vi "7.vi"() -> ()   [LabVIEW 2017]
uses:
  <vilib>/Utility/file.llb/Write Delimited Spreadsheet (DBL).vi
  <vilib>/measure/NI_MABase.lvlib
panel:
  out "Array":dbl[][](array[numeric]) caption="数组"
  out "波形图":waveform(dbl)(graph)
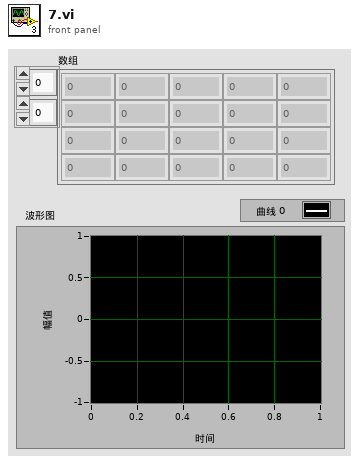
[diagram p1: front panel]
types:
  T1 = enum16{"open", "replace", "create", "open or create", "replace or create", "replace or create with confirmation"}
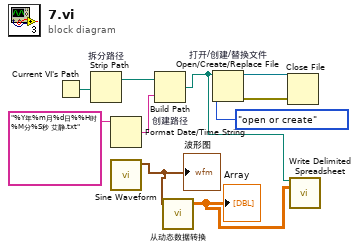
[diagram p0: block diagram]
diagram:
  n1 = Current VI's Path() -> (path=w9:path)
  n2 = Strip Path "拆分路径"(path=w9) -> (stripped path=w7:path)  [unwired: 1 out]
  n3 = Format Date/Time String(time format string (%c)="%Y年%m月%d日%%H时%M分%S秒 艾静.txt" ("时间格式字符串(%c)")) -> (date/time string=w8:string)  [unwired: 2 in]
  n4 = call <vilib>:"Sine Waveform.vi"() -> ("signal out"=w5:waveform(dbl))  [unwired: 10 in, 1 out]
  "波形图" <- w5
  n5 = Build Path "创建路径"(base path=w7, name or relative path=w8) -> (appended path=w3:path)
  n6 = call "从动态数据转换"("Dynamic Data Type"=w5) -> ("Array"=w4:dbl[][])  [unwired: 3 in]
  "Array" <- w4
  n7 = Open/Create/Replace File "打开/创建/替换文件"(file path (use dialog)=w3, operation (0:open)=T1."open or create" ("操作(0:open)")) -> (refnum out=w2:refnum<file>, error out=w1:errorcluster)  [unwired: 4 in, 1 out]
  n8 = Close File(refnum=w2, error in=w1) -> ()  [unwired: 2 out]
  n9 = call-poly <vilib>:"Write Delimited Spreadsheet.vi"("file path (dialog if empty)"=w3, "2D data"=w4) -> ()  [unwired: 12 in, 2 out]
